vi "Main.vi"() -> ()   [LabVIEW 2015, in "Control.lvlib"]
doc: "This template is based off of the Queued Message Handler design pattern and the Queued Message Handler project template that ships with LabVIEW.\n\nThe main difference is that the queue is private to this module and communication between modules is performed via Broadcast and Request events.\n\nRequest events are wrapped in public API methods and are handled in the Event Handling Loop (EHL) of this VI. Any module can register for Broadcast events sent by this module. The EHL generates messages based on user interface actions.\n\nThe Message Handling Loop (MHL) processes messages generated by the EHL, or by other messages. The messages are string values, so new messages can be added easily to the Message Cases case structure in the MHL. Each message cluster can also provide an optional value for Message Data, which is a variant that can be converted to whatever message-specific data is required.\n_____\nBased on Delacor QMH Project Template 4.2.1.64."
uses:
  Control.lvlib
  <vilib>/Delacor/Delacor QMH/Libraries/Module Admin_class/Delacor_lib_QMH_Module Admin.lvclass
  Module Data--cluster.ctl
  <vilib>/Delacor/Delacor QMH/Libraries/Message Queue_class/Delacor_lib_QMH_Message Queue.lvclass/Delacor_lib_QMH_Message Queue.ctl
  Stop Argument--cluster.ctl
  <vilib>/Delacor/Delacor QMH/Libraries/Module Admin_class/Delacor_lib_QMH_Module Admin.lvclass/Delacor_lib_QMH_Module Admin.ctl
  Get Hardware Alias Argument--cluster.ctl
  Get Hardware Alias (Reply Payload)--cluster.ctl
  Start Thermochamber Argument--cluster.ctl
  Start Thermochamber (Reply Payload)--cluster.ctl
  Get Serial Number Argument--cluster.ctl
  Get Serial Number (Reply Payload)--cluster.ctl
  Stop Thermochamber Argument--cluster.ctl
  Stop Thermochamber (Reply Payload)--cluster.ctl
  <vilib>/Utility/miscctls.llb/LVPointTypeDef.ctl
  <vilib>/Delacor/Delacor QMH/Libraries/Message Queue_class/Delacor_lib_QMH_Enqueue Message (Single).vi
  <vilib>/Delacor/Delacor QMH/Libraries/Module Admin_class/Delacor_lib_QMH_Get External Launch.vi
  <vilib>/Utility/error.llb/Error Cluster From Error Code.vi
  <vilib>/ErrorRing/Error Ring.xnode
  <vilib>/Delacor/Delacor QMH/Libraries/Message Queue_class/Delacor_lib_QMH_Message Queue.lvclass
  Thermometer/Thermometer.lvlib
panel:
  in  "Serial Number":string="123ABC-01"
  in  "Start Chamber":bool
  in  "Hardware Alias":string="123ABC-01"
  in  "Simulate MHL Error":bool
  in  "Simulate EHL Error":bool
  out "error out":errorcluster
  in  "Module Admin":refnum<class "Delacor_lib_QMH_Module Admin.lvclass">
  out "Status":string
  # "Control Module\n**This module could be used to control the temperature chambers \nand ensure they're working correctly**"
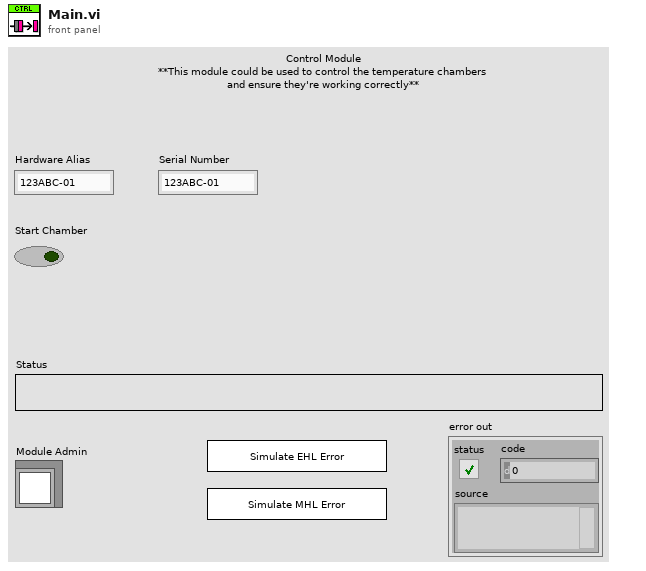
[diagram p1: front panel]
types:
  T1 = typedef "Control.lvlib/Request Events--cluster.ctl" = cluster{"Stop Module":refnum<user-event>, "Show Panel":refnum<user-event>, "Hide Panel":refnum<user-event>, "Get Module Execution Status":refnum<user-event>, "Show Diagram":refnum<user-event>, "Get Hardware Alias":refnum<user-event>, "Start Thermochamber":refnum<user-event>, "Get Serial Number":refnum<user-event>, "Stop Thermochamber":refnum<user-event>}
  T2 = typedef "Thermometer.lvlib/Broadcast Events--cluster.ctl" = cluster{"Module Did Init":refnum<user-event>, "Status Updated":refnum<user-event>, "Error Reported":refnum<user-event>, "Module Did Stop":refnum<user-event>, "Update Module Execution Status":refnum<user-event>}
  T3 = typedef "Control.lvlib/Module Data--cluster.ctl" = cluster{"Status":string}
  T4 = enum32{"invalid lock state", "Not Locked", "Locked (No Password)", "Password-protected"}
  T5 = typedef "Control.lvlib/Stop Argument--cluster.ctl" = cluster{"Origin":string, "Exit via Stop Module Req?":bool, "Wait for Module to stop?":bool}
  T6 = typedef "Control.lvlib/Get Hardware Alias Argument--cluster.ctl" = cluster{"Wait Notifier":refnum<notifier>, "wait for reply":bool}
  T7 = typedef "Control.lvlib/Start Thermochamber Argument--cluster.ctl" = cluster{"Initial Starting Temperature":dbl, "Wait Notifier":refnum<notifier>, "wait for reply":bool}
  T8 = typedef "Control.lvlib/Get Serial Number Argument--cluster.ctl" = cluster{"Wait Notifier":refnum<notifier>, "wait for reply":bool}
  T9 = typedef "Control.lvlib/Stop Thermochamber Argument--cluster.ctl" = cluster{"Wait Notifier":refnum<notifier>, "wait for reply":bool}
  T10 = typedef "LVPointTypeDef.ctl" = cluster{"Horizontal":i16, "Vertical":i16}
  T11 = enum32{"Invalid", "Standard", "Closed", "Hidden", "Minimized", "Maximized"}
  T12 = typedef "Control.lvlib/Get Hardware Alias (Reply Payload)--cluster.ctl" = cluster{"Hardware Alias":string, "Get Hardware Alias_error":errorcluster}
  T13 = typedef "Control.lvlib/Start Thermochamber (Reply Payload)--cluster.ctl" = cluster{"Initialized?":bool, "Start Thermochamber_error":errorcluster}
  T14 = typedef "Control.lvlib/Get Serial Number (Reply Payload)--cluster.ctl" = cluster{"Serial Number":string, "Get Serial Number_error":errorcluster}
  T15 = typedef "Control.lvlib/Stop Thermochamber (Reply Payload)--cluster.ctl" = cluster{"Stop Thermochamber_error":errorcluster}
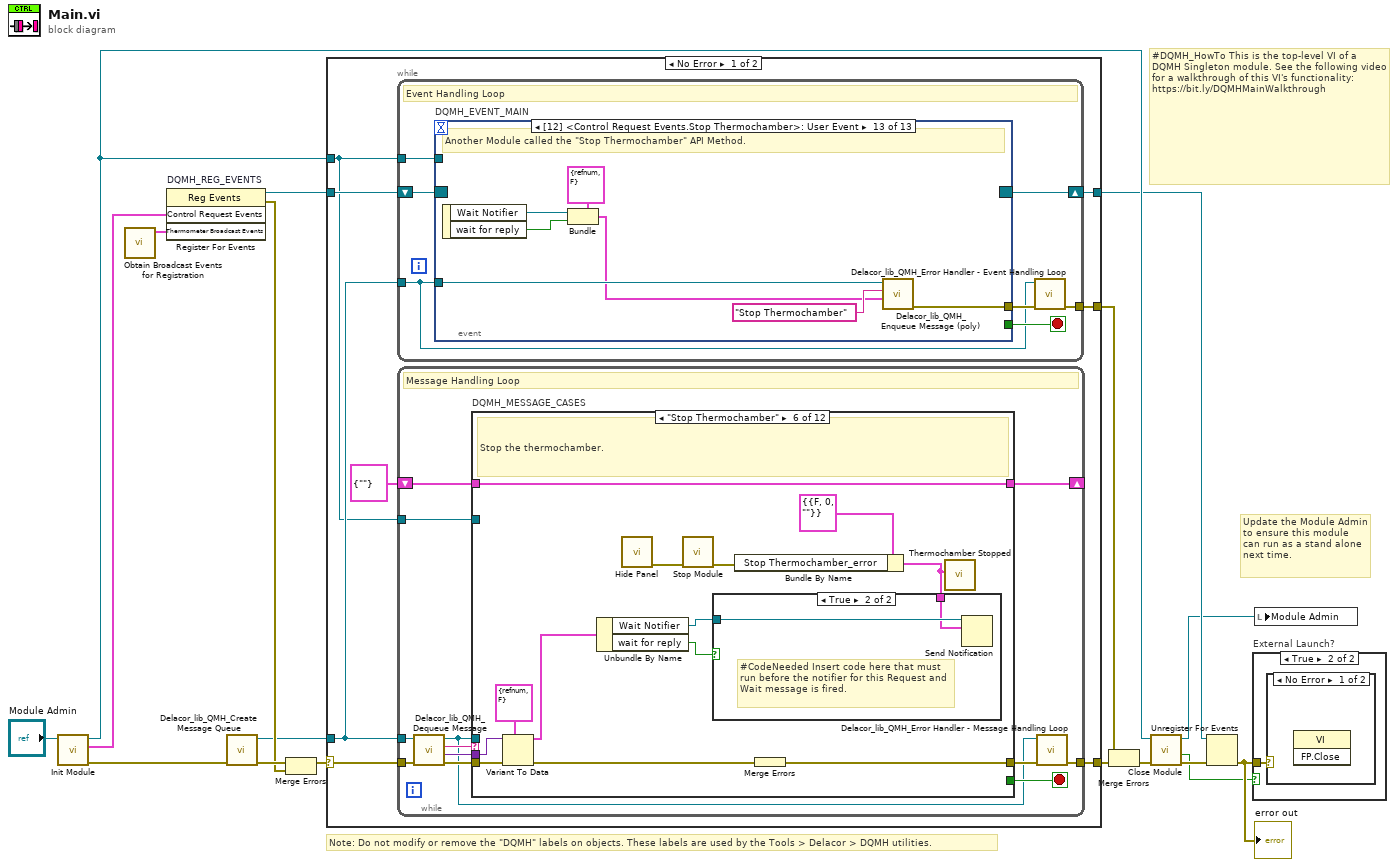
[diagram p0: block diagram]
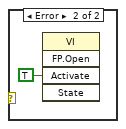
[diagram p3: hidden frame]
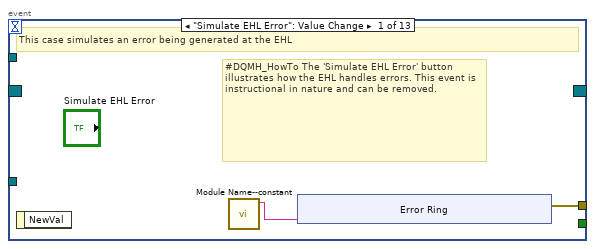
[diagram p4: hidden frame]
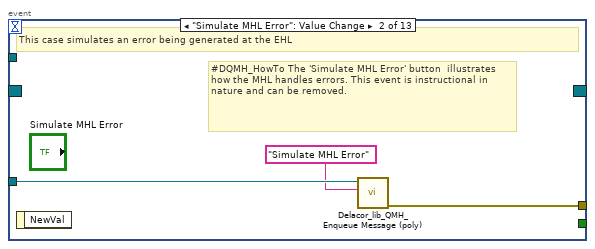
[diagram p5: hidden frame]
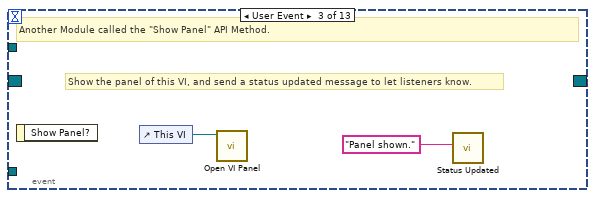
[diagram p6: hidden frame]
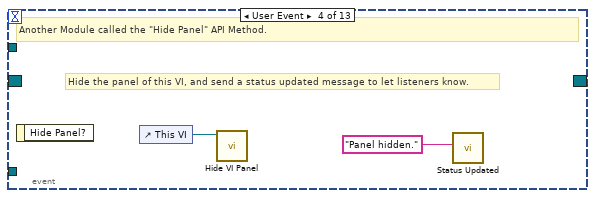
[diagram p7: hidden frame]
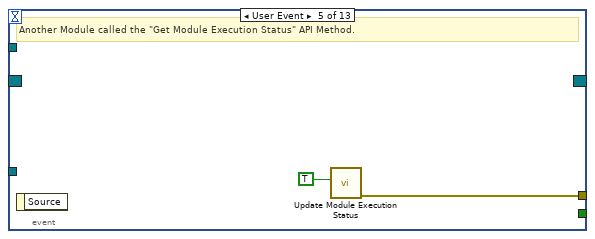
[diagram p8: hidden frame]
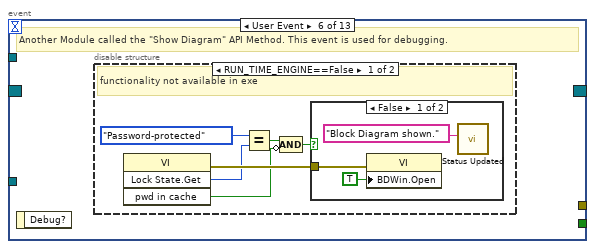
[diagram p9: hidden frame]
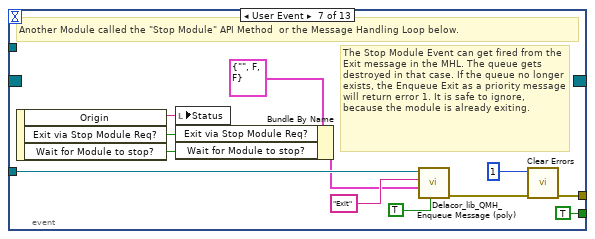
[diagram p12: hidden frame]
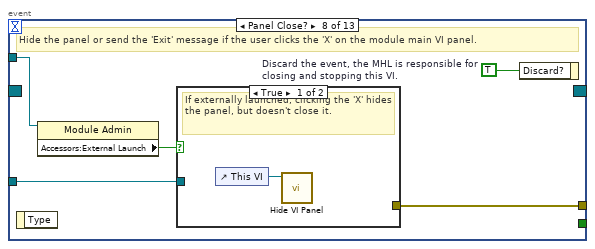
[diagram p13: hidden frame]
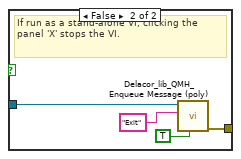
[diagram p14: hidden frame]
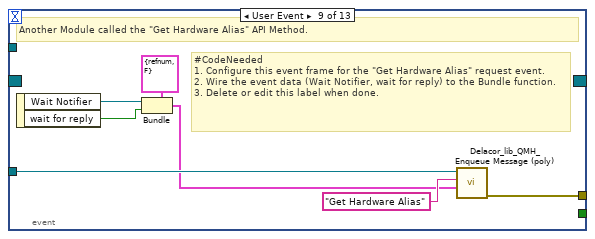
[diagram p15: hidden frame]
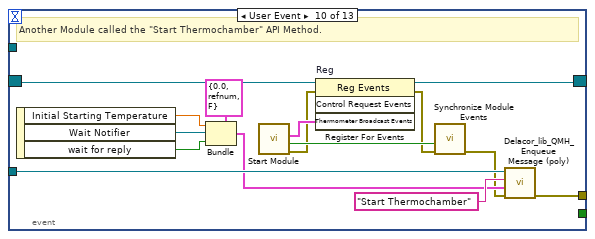
[diagram p16: hidden frame]
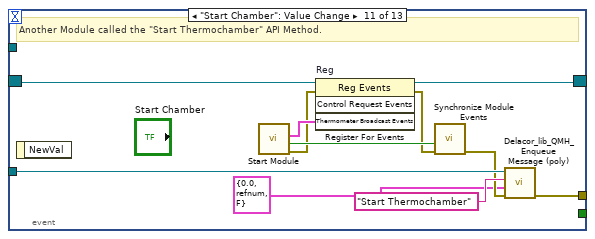
[diagram p17: hidden frame]
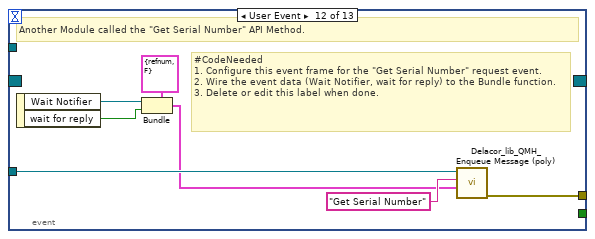
[diagram p18: hidden frame]
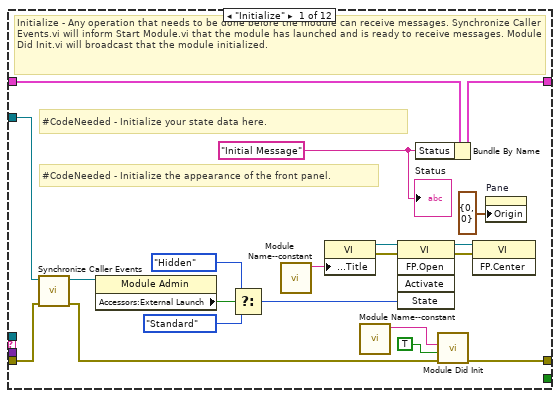
[diagram p19: hidden frame]
diagram:
  # "#DQMH_HowTo This is the top-level VI of a DQMH Singleton module. See the following video for a walkthrough of this VI's functionality: https://bit.ly/DQMHMainWalkthrough"
  # "Note: Do not modify or remove the \"DQMH\" labels on objects. These labels are used by the Tools > Delacor > DQMH utilities."
  # "Update the Module Admin to ensure this module can run as a stand alone next time."
  n1 = call "Init Module.vi"("Singleton Module Admin in"="Module Admin") -> ("error out"=w17:errorcluster, "Control Request Events"=w6:T1, "Singleton Module Admin out"=w9:refnum<class "Delacor_lib_QMH_Module Admin.lvclass">)  [unwired: 8 in]
  n2 = call "Obtain Broadcast Events for Registration.vi"() -> ("Thermometer Broadcast Events"=w1:T2)  [unwired: 9 in, 2 out]
  n3 = register-events "DQMH_REG_EVENTS"(w6, w1) -> (reference out=w7:refnum<event-registration>, error out=w10:errorcluster)  [unwired: 2 in]
  n4 = call <vilib>:"Delacor_lib_QMH_Create Message Queue.vi"("error in (no error)"=w17) -> ("error out"=w12:errorcluster, "Message Queue"=w5:refnum<class "Delacor_lib_QMH_Message Queue.lvclass">)  [unwired: 9 in]
  n5 = Merge Errors(w12, w10) -> (w11:errorcluster)
  n6 = case shown="No Error" w11 {
    selector: w11 -> [w24 w293]
    tunnel: [w26 w293] -> w18
    tunnel: [w23 w290] -> w8
    tunnel: w7 -> [w21 w290]
    tunnel: w5 -> [w20 _]
    tunnel: [w25 _] -> w15
    tunnel: w9 -> [w19 w286]
    frame No Error {
      n7 = while {
        tunnel: w20 -> [w27]
        shift-right: [w30] -> w23
        shift-left: w21 -> [w31]
        tunnel: [w32] -> w25
        tunnel: w19 -> [w28]
        stop <- w29 stop-if-true
        # "Event Handling Loop"
        n8 = event "DQMH_EVENT_MAIN" shown="[12] <Control Request Events.Stop Thermochamber>: User Event" {
          selector: w31 -> [_ _ _ _ _ _ _ _ _ w95 w111 _ _]
          dyn-events: [_ _ _ _ _ _ _ _ _ w96 w112 _ _] -> w30
          timeout: _ -> [_ _ _ _ _ _ _ _ _ _ _ _ _]
          tunnel: [_ _ _ _ _ _ TRUE ("Discard?") _ _ _ _ _ _] -> w29
          tunnel: w27 -> [_ w44 _ _ _ _ w68 w75 w89 w104 w115 w122 w129]
          tunnel: [w35 w45 _ _ w51 _ w71 w77 w85 w100 w113 w118 w125] -> w33
          tunnel: w28 -> [_ _ _ _ _ _ _ w74 _ _ _ _ _]
          event "Simulate EHL Error": Value Change {
            # "#DQMH_HowTo The 'Simulate EHL Error' button  illustrates how the EHL handles errors. This event is instructional in nature and can be removed."
            # "This case simulates an error being generated at the EHL"
            n9 = event-data() -> ()  [unwired: 1 in, 1 out]
            n10 = call "Module Name--constant.vi"() -> ("Module Name"=w34:string)  [unwired: 11 in]
            n11 = xnode "Error Ring"("parameter 0"=w34) -> ("error out"=w35:errorcluster)
          }
          event "Simulate MHL Error": Value Change {
            # "#DQMH_HowTo The 'Simulate MHL Error' button  illustrates how the MHL handles errors. This event is instructional in nature and can be removed."
            # "This case simulates an error being generated at the EHL"
            n12 = event-data() -> ()  [unwired: 1 in, 1 out]
            n13 = call-poly <vilib>:"Delacor_lib_QMH_Enqueue Message (poly).vi"("Message"="Simulate MHL Error", "Message Queue in"=w44) -> ("error out"=w45:errorcluster)  [unwired: 8 in, 1 out]
          }
          event User Event {
            # "Show the panel of this VI, and send a status updated message to let listeners know."
            # "Another Module called the \"Show Panel\" API Method."
            n14 = event-data() -> ()  [unwired: 1 in, 1 out]
            n15 = control-ref of="This VI"() -> (w47:refnum<vi>)
            n16 = call "Open VI Panel.vi"("VI"=w47) -> ()  [unwired: 10 in, 1 out]
            n17 = call "Status Updated.vi"("Status"="Panel shown." ("format string")) -> ()  [unwired: 10 in, 1 out]
          }
          event User Event {
            # "Hide the panel of this VI, and send a status updated message to let listeners know."
            # "Another Module called the \"Hide Panel\" API Method."
            n18 = event-data() -> ()  [unwired: 1 in, 1 out]
            n19 = control-ref of="This VI"() -> (w49:refnum<vi>)
            n20 = call "Hide VI Panel.vi"("VI"=w49) -> ()  [unwired: 10 in, 1 out]
            n21 = call "Status Updated.vi"("Status"="Panel hidden." ("format string")) -> ()  [unwired: 10 in, 1 out]
          }
          event User Event {
            # "Another Module called the \"Get Module Execution Status\" API Method."
            n22 = event-data() -> ()  [unwired: 1 in, 1 out]
            n23 = call "Update Module Execution Status.vi"("Running?"=TRUE) -> ("error out"=w51:errorcluster)  [unwired: 10 in]
          }
          event User Event {
            # "Another Module called the \"Show Diagram\" API Method. This event is used for debugging."
            n24 = event-data() -> ()  [unwired: 1 in, 1 out]
            n25 = disable-structure shown="RUN_TIME_ENGINE==False" {
              frame condition #0 (active) {
                # "functionality not available in exe"
                n26 = invoke class="VI" method="Lock State.Get"() -> (error out=w57:errorcluster, "Get Lock State"=w56:T4, "pwd in cache"=w53:bool)  [unwired: 4 in, 1 out]
                n27 = Equal?(x=T4."Password-protected", y=w56) -> (x = y?=w54:bool)
                n28 = Compound Arithmetic op=AND(w54, invert w53) -> (w52:bool)
                n29 = case shown="False" w52 {
                  tunnel: w57 -> [w60 _]
                  frame False {
                    n30 = property class="VI"(error in=w60, "BDWin.Open"=TRUE ("Block Diagram Window:Open")) -> ()  [unwired: 1 in, 2 out]
                    n31 = call "Status Updated.vi"("Status"="Block Diagram shown." ("format string")) -> ()  [unwired: 10 in, 1 out]
                  }
                  frame True {
                    # "Password-protected VI, and the password is not in the cache. Do not show the diagram."
                  }
                }
              }
              frame condition #1 {
              }
            }
          }
          event User Event {
            # "The Stop Module Event can get fired from the Exit message in the MHL. The queue gets destroyed in that case. If the queue no longer exists, the Enqueue Exit as a priority message will return error 1. It is safe to ignore, because the module is already exiting."
            # "Another Module called the \"Stop Module\" API Method  or the Message Handling Loop below."
            n32 = event-data() -> ("Origin"=w67:string, "Exit via Stop Module Req?"=w63:bool, "Wait for Module to stop?"=w62:bool)  [unwired: 1 in]
            n33 = local write "Status"(w67) -> ()
            n34 = Bundle By Name(cluster=T5 {"Origin"="", "Exit via Stop Module Req?"=FALSE, "Wait for Module to stop?"=FALSE} ("Stop Argument"), "Exit via Stop Module Req?"=w63, "Wait for Module to stop?"=w62) -> (w61:T5)
            n35 = call-poly <vilib>:"Delacor_lib_QMH_Enqueue Message (poly).vi"("Priority Message? (F)"=TRUE, "Message Data"=w61, "Message"="Exit", "Message Queue in"=w68) -> ("error out"=w72:errorcluster)  [unwired: 6 in, 1 out]
            n36 = call <vilib>:"Clear Errors.vi"("error in (no error)"=w72, "specific error code to clear (0: all)"=1) -> ("error out"=w71:errorcluster)  [unwired: 4 in, 1 out]
          }
          event Panel Close? {
            w76 = TRUE  # Discard the event, the MHL is responsible for closing and stopping this VI.
            # "Hide the panel or send the 'Exit' message if the user clicks the 'X' on the module main VI panel."
            n37 = event-data() -> ()  [unwired: 1 in, 1 out]
            n38 = property class="Module Admin"(reference=w74) -> ("Accessors:External Launch"=w73:bool)  [unwired: 1 in, 2 out]
            n39 = case shown="True" w73 {
              tunnel: w75 -> [_ w81]
              tunnel: [_ w82] -> w77
              frame True {
                # "If externally launched, clicking the 'X' hides the panel, but doesn't close it."
                n40 = control-ref of="This VI"() -> (w78:refnum<vi>)
                n41 = call "Hide VI Panel.vi"("VI"=w78) -> ()  [unwired: 10 in, 1 out]
              }
              frame False {
                # "If run as a stand-alone VI, clicking the panel 'X' stops the VI."
                n42 = call-poly <vilib>:"Delacor_lib_QMH_Enqueue Message (poly).vi"("Priority Message? (F)"=TRUE, "Message"="Exit", "Message Queue in"=w81) -> ("error out"=w82:errorcluster)  [unwired: 7 in, 1 out]
              }
            }
            n43 = event-data("Discard?"=w76) -> ()  [unwired: 1 in, 1 out]
          }
          event User Event {
            # "#CodeNeeded\n1. Configure this event frame for the \"Get Hardware Alias\" request event.\n2. Wire the event data (Wait Notifier, wait for reply) to the Bundle function.\n3. Delete or edit this label when done."
            # "Another Module called the \"Get Hardware Alias\" API Method."
            n44 = event-data() -> ("Wait Notifier"=w84:refnum<notifier>, "wait for reply"=w83:bool)  [unwired: 1 in]
            n45 = Bundle(cluster=T6 {"Wait Notifier"=refnum, "wait for reply"=FALSE} ("Get Hardware Alias Argument"), "Wait Notifier"=w84, "wait for reply"=w83) -> (w86:T6)
            n46 = call-poly <vilib>:"Delacor_lib_QMH_Enqueue Message (poly).vi"("Message Data"=w86, "Message"="Get Hardware Alias", "Message Queue in"=w89) -> ("error out"=w85:errorcluster)  [unwired: 7 in, 1 out]
          }
          event User Event {
            # "Another Module called the \"Start Thermochamber\" API Method."
            n47 = event-data() -> ("Initial Starting Temperature"=w99:dbl, "Wait Notifier"=w98:refnum<notifier>, "wait for reply"=w97:bool)  [unwired: 1 in]
            n48 = Bundle(cluster=T7 {"Initial Starting Temperature"=0.0, "Wait Notifier"=refnum, "wait for reply"=FALSE} ("Start Thermochamber Argument"), "Initial Starting Temperature"=w99, "Wait Notifier"=w98, "wait for reply"=w97) -> (w101:T7)
            n49 = call "Start Module.vi"() -> ("error out"=w92:errorcluster, "Wait for Event Sync?"=w93:bool, "Thermometer Broadcast Events"=w94:T2)  [unwired: 8 in, 1 out]
            n50 = register-events "Reg"(reference=w95, error in=w92, w94) -> (reference out=w96:refnum<event-registration>, error out=w91:errorcluster)  [unwired: 1 in]
            n51 = call "Synchronize Module Events.vi"("error in (no error)"=w91, "Wait for Event Sync?"=w93) -> ("error out"=w90:errorcluster)  [unwired: 9 in]
            n52 = call-poly <vilib>:"Delacor_lib_QMH_Enqueue Message (poly).vi"("error in (no error)"=w90, "Message Data"=w101, "Message"="Start Thermochamber", "Message Queue in"=w104) -> ("error out"=w100:errorcluster)  [unwired: 6 in, 1 out]
          }
          event "Start Chamber": Value Change {
            # "Another Module called the \"Start Thermochamber\" API Method."
            n53 = event-data() -> ()  [unwired: 1 in, 1 out]
            n54 = call "Start Module.vi"() -> ("error out"=w108:errorcluster, "Wait for Event Sync?"=w109:bool, "Thermometer Broadcast Events"=w110:T2)  [unwired: 8 in, 1 out]
            n55 = register-events "Reg"(reference=w111, error in=w108, w110) -> (reference out=w112:refnum<event-registration>, error out=w107:errorcluster)  [unwired: 1 in]
            n56 = call "Synchronize Module Events.vi"("error in (no error)"=w107, "Wait for Event Sync?"=w109) -> ("error out"=w106:errorcluster)  [unwired: 9 in]
            n57 = call-poly <vilib>:"Delacor_lib_QMH_Enqueue Message (poly).vi"("error in (no error)"=w106, "Message Data"=T7 {"Initial Starting Temperature"=0.0, "Wait Notifier"=refnum, "wait for reply"=FALSE} ("Start Thermochamber Argument"), "Message"="Start Thermochamber", "Message Queue in"=w115) -> ("error out"=w113:errorcluster)  [unwired: 6 in, 1 out]
          }
          event User Event {
            # "#CodeNeeded\n1. Configure this event frame for the \"Get Serial Number\" request event.\n2. Wire the event data (Wait Notifier, wait for reply) to the Bundle function.\n3. Delete or edit this label when done."
            # "Another Module called the \"Get Serial Number\" API Method."
            n58 = event-data() -> ("Wait Notifier"=w117:refnum<notifier>, "wait for reply"=w116:bool)  [unwired: 1 in]
            n59 = Bundle(cluster=T8 {"Wait Notifier"=refnum, "wait for reply"=FALSE} ("Get Serial Number Argument"), "Wait Notifier"=w117, "wait for reply"=w116) -> (w119:T8)
            n60 = call-poly <vilib>:"Delacor_lib_QMH_Enqueue Message (poly).vi"("Message Data"=w119, "Message"="Get Serial Number", "Message Queue in"=w122) -> ("error out"=w118:errorcluster)  [unwired: 7 in, 1 out]
          }
          event User Event {
            # "Another Module called the \"Stop Thermochamber\" API Method."
            n61 = event-data() -> ("Wait Notifier"=w124:refnum<notifier>, "wait for reply"=w123:bool)  [unwired: 1 in]
            n62 = Bundle(cluster=T9 {"Wait Notifier"=refnum, "wait for reply"=FALSE} ("Stop Thermochamber Argument"), "Wait Notifier"=w124, "wait for reply"=w123) -> (w126:T9)
            n63 = call-poly <vilib>:"Delacor_lib_QMH_Enqueue Message (poly).vi"("Message Data"=w126, "Message"="Stop Thermochamber", "Message Queue in"=w129) -> ("error out"=w125:errorcluster)  [unwired: 7 in, 1 out]
          }
        }
        n64 = call-dynamic "Delacor_lib_QMH_Error Handler - Event Handling Loop.vi"("error in (no error)"=w33, "Message Queue in"=w27) -> ("dup error in"=w32:errorcluster)  [unwired: 8 in, 1 out]
      }
      n65 = while {
        tunnel: w20 -> [w132]
        shift-right: [w136] -> _
        shift-left: T3 {"Status"=""} ("Data Cluster") -> [w137]
        tunnel: w24 -> [w140]
        tunnel: [w138] -> w26
        tunnel: w19 -> [w130]
        stop <- w135 stop-if-true
        # "Message Handling Loop"
        n66 = call-dynamic "Delacor_lib_QMH_Dequeue Message.vi"("error in (no error)"=w140, "Message Queue in"=w132) -> ("error out"=w139:errorcluster, "Message Data"=w133:variant, "Message"=w134:string, "Message Queue out"=w131:refnum<class "Delacor_lib_QMH_Message Queue.lvclass">)  [unwired: 6 in]
        n67 = case "DQMH_MESSAGE_CASES" shown="\"Stop Thermochamber\"" w134 {
          selector: w134 -> [_ _ _ _ _ _ _ _ _ _ _ w273]
          tunnel: w131 -> [_ _ _ _ _ _ _ _ _ w243 w265 _]
          tunnel: w139 -> [w159 w163 w175 w192 w206 w221 w226 w228 w233 w250 w271 w275]
          tunnel: [w157 w163 w165 w182 w196 w211 w225 w228 w232 w246 w268 w276] -> w141
          tunnel: w137 -> [w148 w162 w174 w191 w205 w220 w224 w227 w230 w245 w264 w274]
          tunnel: [w147 w162 w174 w191 w205 w220 w224 w227 w230 w245 w264 w274] -> w136
          tunnel: [_ _ _ _ _ _ _ _ _ _ w263 _] -> w135
          tunnel: w133 -> [_ _ w172 w189 w203 w218 _ _ _ w244 w262 _]
          tunnel: w130 -> [w149 _ _ _ _ _ _ _ _ w242 w257 _]
          frame "Initialize" {
            w142 = "Initial Message" ("Initial Message")
            # "#CodeNeeded - Initialize the appearance of the front panel."
            # "#CodeNeeded - Initialize your state data here."
            # "Initialize - Any operation that needs to be done before the module can receive messages. Synchronize Caller Events.vi will inform Start Module.vi that the module has launched and is ready to receive messages. Module Did Init.vi will broadcast that the module initialized."
            n68 = call "Synchronize Caller Events.vi"("error in (no error)"=w159, "Singleton Module Admin in"=w149) -> ("error out"=w158:errorcluster, "Singleton Module Admin out"=w144:refnum<class "Delacor_lib_QMH_Module Admin.lvclass">)  [unwired: 8 in]
            n69 = property class="Module Admin"(reference=w144) -> ("Accessors:External Launch"=w153:bool)  [unwired: 1 in, 2 out]
            n70 = Select(t=T11."Hidden" ("State"), s=w153, f=T11."Standard" ("State")) -> (s? t:f=w150:T11)
            n71 = call "Module Name--constant.vi"() -> ("Module Name"=w156:string)  [unwired: 11 in]
            n72 = property class="VI"("Front Panel.Title"=w156) -> (reference out=w155:refnum<vi>, error out=w161:errorcluster)  [unwired: 2 in]
            n73 = call "Module Name--constant.vi"() -> ("Module Name"=w145:string)  [unwired: 11 in]
            n74 = invoke class="VI" method="FP.Open"(reference=w155, error in=w161, "State"=w150) -> (reference out=w154:refnum<vi>, error out=w160:errorcluster)  [unwired: 2 in, 3 out]
            n75 = Bundle By Name(cluster=w148, "Status"=w142) -> (w147:T3)
            n76 = call "Module Did Init.vi"("error in (no error)"=w158, "Initialized?"=TRUE, "Origin"=w145) -> ("error out"=w157:errorcluster)  [unwired: 8 in]
            n77 = invoke class="VI" method="FP.Center"(reference=w154, error in=w160) -> ()  [unwired: 1 in, 3 out]
            n78 = property on="Pane" class="Pane"("Origin"=T10 {"Horizontal"=0, "Vertical"=0}) -> ()  [unwired: 2 in, 2 out]
            "Status" <- w142
          }
          frame "--- Module Specific ---" {
            # "Separator -- The following cases handle messages specific to this Module."
          }
          frame "Get Hardware Alias" {
            # "This will return the hardware alias."
            n79 = Variant To Data(error in=w175, type=T6 {"Wait Notifier"=refnum, "wait for reply"=FALSE} ("Get Hardware Alias Argument"), Variant=w172) -> (data=w170:T6, error out=w173:errorcluster)
            n80 = Unbundle By Name(w170) -> ("Wait Notifier"=w169:refnum<notifier>, "wait for reply"=w168:bool)
            n81 = Merge Errors(w173) -> (w165:errorcluster)
            n82 = Bundle By Name(cluster=T12 {"Hardware Alias"="", "Get Hardware Alias_error"={"status"=FALSE, "code"=0, "source"=""}} ("Get Hardware Alias (Reply Payload)"), "Hardware Alias"="Hardware Alias") -> (w167:T12)
            n83 = case shown="True" w168 {
              tunnel: w169 -> [_ w177]
              tunnel: w167 -> [_ w176]
              frame False {
              }
              frame True {
                n84 = Send Notification(notification=w176, notifier=w177) -> ()  [unwired: 1 in, 2 out]
              }
            }
          }
          frame "Start Thermochamber" {
            # "Start the thermochamber."
            n85 = Variant To Data(error in=w192, type=T7 {"Initial Starting Temperature"=0.0, "Wait Notifier"=refnum, "wait for reply"=FALSE} ("Start Thermochamber Argument"), Variant=w189) -> (data=w187:T7, error out=w190:errorcluster)
            n86 = Unbundle By Name(w187) -> ("Initial Starting Temperature"=w180:dbl, "Wait Notifier"=w186:refnum<notifier>, "wait for reply"=w185:bool)
            n87 = call "Show Panel.vi"() -> ("error out"=w178:errorcluster)  [unwired: 11 in]
            n88 = call "Start.vi"("error in (no error)"=w178, "Starting Temperature"=w180) -> ("error out"=w179:errorcluster)  [unwired: 9 in]
            n89 = Merge Errors(w190) -> (w182:errorcluster)
            n90 = Bundle By Name(cluster=T13 {"Initialized?"=FALSE, "Start Thermochamber_error"={"status"=FALSE, "code"=0, "source"=""}} ("Start Thermochamber (Reply Payload)"), "Initialized?"=TRUE, "Start Thermochamber_error"=w179) -> (w184:T13)
            n91 = case shown="True" w185 {
              tunnel: w186 -> [_ w194]
              tunnel: w184 -> [_ w193]
              frame False {
              }
              frame True {
                n92 = Send Notification(notification=w193, notifier=w194) -> ()  [unwired: 1 in, 2 out]
              }
            }
            n93 = call "Thermochamber Started.vi"("Reply Payload"=w184) -> ()  [unwired: 10 in, 1 out]
          }
          frame "Get Serial Number" {
            # "Return Serial Number."
            n94 = Variant To Data(error in=w206, type=T8 {"Wait Notifier"=refnum, "wait for reply"=FALSE} ("Get Serial Number Argument"), Variant=w203) -> (data=w201:T8, error out=w204:errorcluster)
            n95 = Unbundle By Name(w201) -> ("Wait Notifier"=w200:refnum<notifier>, "wait for reply"=w199:bool)
            n96 = Merge Errors(w204) -> (w196:errorcluster)
            n97 = Bundle By Name(cluster=T14 {"Serial Number"="", "Get Serial Number_error"={"status"=FALSE, "code"=0, "source"=""}} ("Get Serial Number (Reply Payload)"), "Serial Number"="Serial Number") -> (w198:T14)
            n98 = case shown="True" w199 {
              tunnel: w200 -> [_ w208]
              tunnel: w198 -> [_ w207]
              frame False {
              }
              frame True {
                n99 = Send Notification(notification=w207, notifier=w208) -> ()  [unwired: 1 in, 2 out]
              }
            }
          }
          frame "Stop Thermochamber" {
            # "Stop the thermochamber."
            n100 = Variant To Data(error in=w221, type=T9 {"Wait Notifier"=refnum, "wait for reply"=FALSE} ("Stop Thermochamber Argument"), Variant=w218) -> (data=w216:T9, error out=w219:errorcluster)
            n101 = Unbundle By Name(w216) -> ("Wait Notifier"=w215:refnum<notifier>, "wait for reply"=w214:bool)
            n102 = call "Hide Panel.vi"() -> ("error out"=w210:errorcluster)  [unwired: 11 in]
            n103 = call "Stop Module.vi"("error in (no error)"=w210) -> ("error out"=w209:errorcluster)  [unwired: 10 in]
            n104 = Bundle By Name(cluster=T15 {"Stop Thermochamber_error"={"status"=FALSE, "code"=0, "source"=""}} ("Stop Thermochamber (Reply Payload)"), "Stop Thermochamber_error"=w209) -> (w213:T15)
            n105 = case shown="True" w214 {
              tunnel: w215 -> [_ w223]
              tunnel: w213 -> [_ w222]
              frame False {
              }
              frame True {
                # "#CodeNeeded Insert code here that must run before the notifier for this Request and Wait message is fired."
                n106 = Send Notification(notification=w222, notifier=w223) -> ()  [unwired: 1 in, 2 out]
              }
            }
            n107 = Merge Errors(w219) -> (w211:errorcluster)
            n108 = call "Thermochamber Stopped.vi"("Reply Payload"=w213) -> ()  [unwired: 10 in, 1 out]
          }
          frame "---Copy This Frame---" {
            # "Duplicate this frame when creating new messages.  Change this comment in the duplicated frame to describe this message."
            n109 = Merge Errors(w226) -> (w225:errorcluster)
          }
          frame "--- Exit and Error Handling---" {
            # "Separator - The following cases handle errors and exit messages."
          }
          frame "Simulate MHL Error" {
            # "#DQMH_HowTo The 'Simulate MHL Error' button  illustrates how the MHL handles errors. This event is instructional in nature and can be removed."
            # "Simulate an error occurring at the MHL"
            n110 = call "Module Name--constant.vi"() -> ("Module Name"=w229:string)  [unwired: 11 in]
            n111 = xnode "Error Ring"("parameter 0"=w229) -> ("error out"=w231:errorcluster)
            n112 = Merge Errors(w233, w231) -> (w232:errorcluster)
          }
          frame "Error" {
            # "#CodeRecommended - If you ever change the name of this \"Error\" message, you'll need to update the name in the Check Loop Error.vi as well."
            # "#CodeRecommended - If the module is running in standalone mode (External Launch = FALSE), this code will pop up an error dialog and call the 'Exit' message if an error occurs. Add more fine-grained error handling here."
            # "Error - Check the error message data and respond accordingly. This message is sent by the \"Error Handler\" VIs at the end of each loop in this application."
            n113 = property class="Module Admin"(reference=w242) -> ("Accessors:External Launch"=w241:bool)  [unwired: 1 in, 2 out]
            n114 = Variant To Data(error in=w250, type=errorcluster {"status"=FALSE, "code"=0, "source"=""} ("error constant"), Variant=w244) -> (data=w251:errorcluster, error out=w248:errorcluster)
            n115 = call "Error Reported.vi"("Error"=w251) -> ()  [unwired: 10 in, 1 out]
            n116 = case shown="False" w241 {
              tunnel: [w256 _] -> w247
              tunnel: w243 -> [w254 _]
              tunnel: w251 -> [w255 _]
              frame False {
                # "If the module is running standalone, then pop up an error dialog and call the \"Exit\" message."
                n117 = call <vilib>:"Simple Error Handler.vi"("error in (no error)"=w255) -> ()  [unwired: 4 in, 5 out]
                n118 = call-poly <vilib>:"Delacor_lib_QMH_Enqueue Message (poly).vi"("Priority Message? (F)"=TRUE, "Message"="Exit", "Message Queue in"=w254) -> ("error out"=w256:errorcluster)  [unwired: 7 in, 1 out]
              }
              frame True {
                # "If the module was launched externally, calling the Error Reported broadcast VI is the only action performed by the \"Error\" message. The module's caller can then process the error appropriately."
              }
            }
            n119 = Merge Errors(w248, w247) -> (w246:errorcluster)
            n120 = local write "error out"(w246) -> ()
          }
          frame "Exit" {
            w261 = 91  # 91: not all Exit messages will have an argument
            w263 = TRUE  # Stop the VI
            # "Release the message queue reference"
            # "#CodeNeeded - Add any required cleanup code here"
            # "Exit - Exit the application."
            n121 = Variant To Data(error in=w271, type=T5 {"Origin"="", "Exit via Stop Module Req?"=FALSE, "Wait for Module to stop?"=FALSE} ("Stop Argument"), Variant=w262) -> (data=w259:T5, error out=w267:errorcluster)
            n122 = call <vilib>:"Clear Errors.vi"("error in (no error)"=w267, "specific error code to clear (0: all)"=w261) -> ("error out"=w270:errorcluster)  [unwired: 4 in, 1 out]
            n123 = control-ref of="This VI"() -> (w258:refnum<vi>)
            n124 = call-dynamic "Delacor_lib_QMH_Release Message Queue.vi"("error in (no error)"=w270, "Message Queue"=w265) -> ("error out"=w269:errorcluster)  [unwired: 9 in]
            n125 = call "Handle Exit.vi"("Stop Argument"=w259, "Admin in"=w257, "VI reference"=w258) -> ("error out"=w266:errorcluster)  [unwired: 7 in, 1 out]
            n126 = Merge Errors(w269, w266) -> (w268:errorcluster)
            n127 = call "Stop Module.vi"() -> ()  [unwired: 11 in, 1 out]
          }
          frame Default {
            # "'Default' case only runs if there is a message that isn't defined in any of the other cases.  Output a programming error."
            n128 = call "Module Name--constant.vi"() -> ("Module Name"=w272:string)  [unwired: 11 in]
            n129 = xnode "Error Ring"("parameter 0"=w273, "parameter 1"=w272) -> ("error out"=w277:errorcluster)
            n130 = Merge Errors(w275, w277) -> (w276:errorcluster)
          }
        }
        n131 = call-dynamic "Delacor_lib_QMH_Error Handler - Message Handling Loop.vi"("error in (no error)"=w141, "Message Queue in"=w131) -> ("dup error in"=w138:errorcluster)  [unwired: 8 in, 1 out]
      }
    }
    frame Error {
      # "Synchronize Caller Events.vi will inform Start Module.vi that the module has launched and will let the code calling Start Module.vi register for broadcasts and would permit the caller receive the broadcast that an error occurred at launch time."
      n132 = call "Synchronize Caller Events.vi"("Singleton Module Admin in"=w286) -> ("error out"=w291:errorcluster)  [unwired: 9 in, 1 out]
      n133 = call "Module Name--constant.vi"() -> ("Module Name"=w289:string)  [unwired: 11 in]
      n134 = Format Into String(format string="An error occurred during initialization. %s is no longer running.", w289) -> (resulting string=w287:string)  [unwired: 2 in, 1 out]
      n135 = Merge Errors(w293, w291) -> (w292:errorcluster)
      n136 = call "Error Reported.vi"("Additional Information"=w287, "Error"=w292) -> ()  [unwired: 9 in, 1 out]
    }
  }
  n137 = Merge Errors(w15, w18) -> (w14:errorcluster)
  n138 = call "Close Module.vi"("error in (no error)"=w14, "Module Admin in"=w9) -> ("error out"=w16:errorcluster, "External Launch"=w2:bool, "Module Admin out"=w3:refnum<class "Delacor_lib_QMH_Module Admin.lvclass">)  [unwired: 7 in]
  n139 = Unregister For Events(event registration refnum=w8, error in=w16) -> (error out=w13:errorcluster)
  "error out" <- w13
  n140 = case "External Launch?" shown="True" w2 {
    tunnel: w13 -> [_ w294]
    frame False {
    }
    frame True {
      n141 = case shown="No Error" w294 {
        frame No Error {
          n142 = invoke class="VI" method="FP.Close"() -> ()  [unwired: 3 in, 3 out]
        }
        frame Error {
          n143 = invoke class="VI" method="FP.Open"("Activate"=TRUE ("Activate?")) -> ()  [unwired: 4 in, 5 out]
        }
      }
    }
  }
  n144 = local write "Module Admin"(w3) -> ()
